vi "Serial Data Communication Event Case.vi"() -> ()   [LabVIEW 2020]
uses:
  <vilib>/Instr/_visa.llb/VISA Configure Serial Port (Instr).vi
panel:
  out "?":u32
  in  "Samples":u16
  out "Waveform Chart":i32(graph)
  in  "Send":bool
  in  "Send":bool
  in  "Channel":u8
  out "Monitor":string
  in  "START":bool
  in  "VISA resource name":refnum<visa-resource-name>
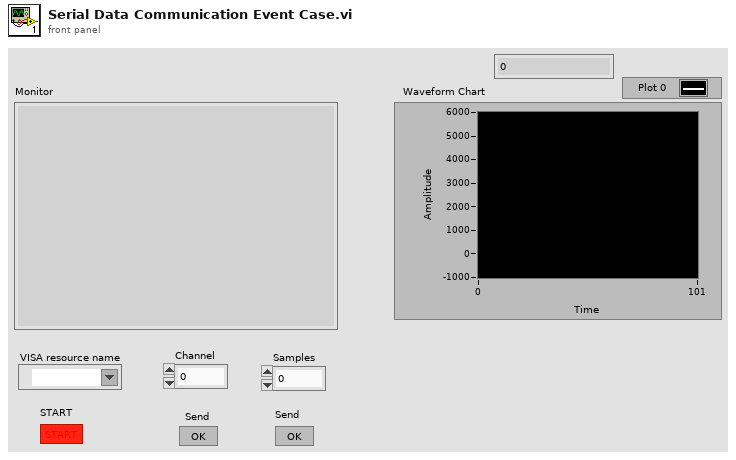
[diagram p1: front panel]
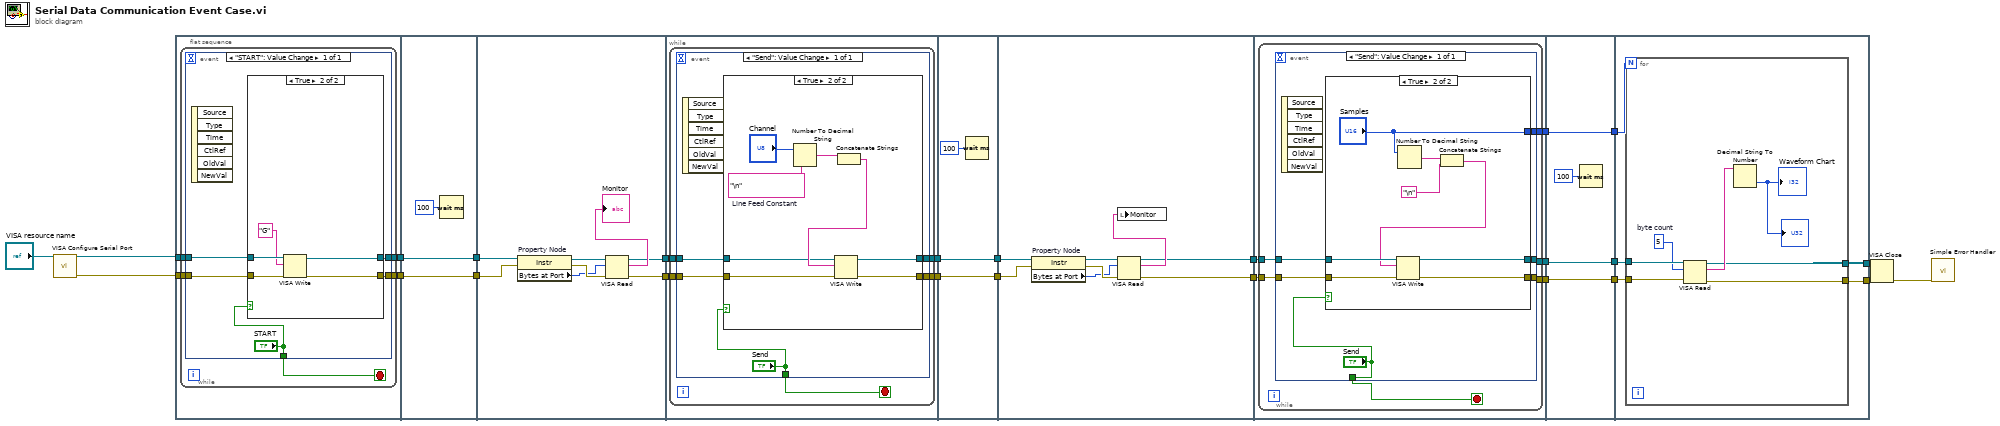
[diagram p0: block diagram]
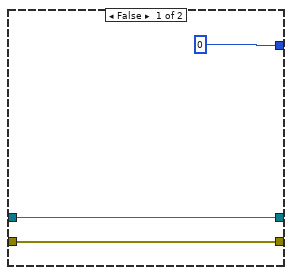
[diagram p4: hidden frame]
diagram:
  n1 = call-poly "VISA Configure Serial Port"("VISA resource name"="VISA resource name") -> ("VISA resource name out"=w23:refnum<visa-resource-name>, "error out"=w22:errorcluster)  [unwired: 13 in]
  n2 = flat-sequence {
    tunnel: w23 -> [w28]
    tunnel: w22 -> [w27]
    tunnel: [w26] -> w20
    tunnel: [w25] -> w18
    tunnel: [w47] -> w21
    tunnel: w20 -> [w47]
    tunnel: [w46] -> w19
    tunnel: w18 -> [w46]
    tunnel: w21 -> [w56]
    tunnel: w19 -> [w55]
    tunnel: [w50] -> w17
    tunnel: [w49] -> w16
    tunnel: w17 -> [w60]
    tunnel: w16 -> [w59]
    tunnel: [w58] -> w14
    tunnel: [w57] -> w12
    tunnel: [w82] -> w15
    tunnel: w14 -> [w82]
    tunnel: [w81] -> w13
    tunnel: w12 -> [w81]
    tunnel: w15 -> [w91]
    tunnel: w13 -> [w90]
    tunnel: [w85] -> w11
    tunnel: [w84] -> w10
    tunnel: w11 -> [w96]
    tunnel: w10 -> [w95]
    tunnel: [w94] -> w9
    tunnel: [w93] -> w6
    tunnel: [w92] -> w4
    tunnel: w9 -> [w122]
    tunnel: [w122] -> w8
    tunnel: [w121] -> w7
    tunnel: w6 -> [w121]
    tunnel: [w120] -> w5
    tunnel: w4 -> [w120]
    tunnel: w8 -> [w128]
    tunnel: w7 -> [w127]
    tunnel: w5 -> [w126]
    tunnel: [w125] -> w3
    tunnel: [w124] -> w2
    frame #0 {
      n3 = while {
        tunnel: w28 -> [w32]
        tunnel: w27 -> [w31]
        tunnel: [w30] -> w26
        tunnel: [w29] -> w25
        stop <- w33 stop-if-true
        n4 = event shown="[0] \"START\": Value Change" {
          selector: _ -> [_]
          dyn-events: _ -> [_]
          timeout: _ -> [_]
          tunnel: ["START"] -> w33
          tunnel: w32 -> [w37]
          tunnel: w31 -> [w36]
          tunnel: [w35] -> w30
          tunnel: [w34] -> w29
          event "START": Value Change {
            n5 = event-data() -> ()  [unwired: 1 in, 6 out]
            n6 = case shown="True" "START" {
              tunnel: w37 -> [w40 w45]
              tunnel: w36 -> [w39 w44]
              tunnel: [w40 w42] -> w35
              tunnel: [w39 w41] -> w34
              frame False {
              }
              frame True {
                n7 = VISA Write(VISA resource name=w45, write buffer="G", error in (no error)=w44) -> (VISA resource name out=w42:refnum<visa-resource-name>, error out=w41:errorcluster)  [unwired: 1 out]
              }
            }
          }
        }
      }
    }
    frame #1 {
      n8 = Wait (ms)(milliseconds to wait=u32 100) -> ()  [unwired: 1 out]
    }
    frame #2 {
      n9 = property on="Property Node" class="Instr"(reference=w56, error in=w55) -> (reference out=w54:refnum<visa-resource-name>, error out=w53:errorcluster, "Bytes at Port"=w52:u32)
      n10 = VISA Read(VISA resource name=w54, byte count=w52, error in (no error)=w53) -> (VISA resource name out=w50:refnum<visa-resource-name>, read buffer=→"Monitor":string, error out=w49:errorcluster)  [unwired: 1 out]
    }
    frame #3 {
      n11 = while {
        tunnel: w60 -> [w64]
        tunnel: w59 -> [w63]
        tunnel: [w62] -> w58
        tunnel: [w61] -> w57
        stop <- w65 stop-if-true
        n12 = event shown="[0] \"Send\": Value Change" {
          selector: _ -> [_]
          dyn-events: _ -> [_]
          timeout: _ -> [_]
          tunnel: ["Send"] -> w65
          tunnel: w64 -> [w69]
          tunnel: w63 -> [w68]
          tunnel: [w67] -> w62
          tunnel: [w66] -> w61
          event "Send": Value Change {
            n13 = event-data() -> ()  [unwired: 1 in, 6 out]
            n14 = case shown="True" "Send" {
              tunnel: w69 -> [w72 w76]
              tunnel: w68 -> [w71 w75]
              tunnel: [w72 w74] -> w67
              tunnel: [w71 w73] -> w66
              frame False {
              }
              frame True {
                w78 = "\n"  # Line Feed Constant
                n15 = Number To Decimal String(number="Channel") -> (decimal integer string=w79:string)  [unwired: 1 in]
                n16 = Concatenate Strings "Concatenate Strings"(w79, w78) -> (w77:string)
                n17 = VISA Write(VISA resource name=w76, write buffer=w77, error in (no error)=w75) -> (VISA resource name out=w74:refnum<visa-resource-name>, error out=w73:errorcluster)  [unwired: 1 out]
              }
            }
          }
        }
      }
    }
    frame #4 {
      n18 = Wait (ms)(milliseconds to wait=u32 100) -> ()  [unwired: 1 out]
    }
    frame #5 {
      n19 = property on="Property Node" class="Instr"(reference=w91, error in=w90) -> (reference out=w87:refnum<visa-resource-name>, error out=w89:errorcluster, "Bytes at Port"=w88:u32)
      n20 = VISA Read(VISA resource name=w87, byte count=w88, error in (no error)=w89) -> (VISA resource name out=w85:refnum<visa-resource-name>, read buffer=w86:string, error out=w84:errorcluster)  [unwired: 1 out]
      n21 = local write "Monitor"(w86) -> ()
    }
    frame #6 {
      n22 = while {
        tunnel: w96 -> [w101]
        tunnel: w95 -> [w100]
        tunnel: [w97] -> w94
        tunnel: [w99] -> w93
        tunnel: [w98] -> w92
        stop <- w102 stop-if-true
        n23 = event shown="[0] \"Send\": Value Change" {
          selector: _ -> [_]
          dyn-events: _ -> [_]
          timeout: _ -> [_]
          tunnel: ["Send"] -> w102
          tunnel: w101 -> [w107]
          tunnel: w100 -> [w106]
          tunnel: [w105] -> w99
          tunnel: [w104] -> w98
          tunnel: [w103] -> w97
          event "Send": Value Change {
            n24 = event-data() -> ()  [unwired: 1 in, 6 out]
            n25 = case shown="True" "Send" {
              tunnel: w107 -> [w111 w119]
              tunnel: w106 -> [w110 w118]
              tunnel: [w111 w117] -> w105
              tunnel: [w110 w116] -> w104
              tunnel: [0 "Samples"] -> w103
              frame False {
              }
              frame True {
                n26 = Number To Decimal String(number="Samples") -> (decimal integer string=w113:string)  [unwired: 1 in]
                n27 = Concatenate Strings "Concatenate Strings"(w113, "\n") -> (w112:string)
                n28 = VISA Write(VISA resource name=w119, write buffer=w112, error in (no error)=w118) -> (VISA resource name out=w117:refnum<visa-resource-name>, error out=w116:errorcluster)  [unwired: 1 out]
              }
            }
          }
        }
      }
    }
    frame #7 {
      n29 = Wait (ms)(milliseconds to wait=u32 100) -> ()  [unwired: 1 out]
    }
    frame #8 {
      n30 = for {
        N: w128 -> [_]
        tunnel: w127 -> [w135]
        tunnel: w126 -> [w134]
        tunnel: [w131] -> w125
        tunnel: [w130] -> w124
        w133 = u32 5  # byte count
        n31 = VISA Read(VISA resource name=w135, byte count=w133, error in (no error)=w134) -> (VISA resource name out=w131:refnum<visa-resource-name>, read buffer=w132:string, error out=w130:errorcluster)  [unwired: 1 out]
        n32 = Decimal String To Number(string=w132) -> (number=→"Waveform Chart" →"?":i32)  [unwired: 2 in, 1 out]
      }
    }
  }
  n33 = VISA Close(VISA resource name=w3, error in (no error)=w2) -> (error out=w1:errorcluster)
  n34 = call <vilib>:"Simple Error Handler.vi"("error in (no error)"=w1) -> ()  [unwired: 4 in, 5 out]
